vi "Actor Core.vi"(8 "error in":errorcluster, 11 "Panel Manager Controller.lvclass":refnum<class "Panel Manager Controller.lvclass">) -> (0 "error out":errorcluster, 3 "Actor out":refnum<class "Actor.lvclass">)   [LabVIEW 2015, in "Panel Manager Controller.lvclass"]
doc: "(<B>Filename</B>: Actor Framework.lvlib:Actor.lvclass:Actor Core.vi)\n\nReceives messages to the actor, reacts to them, and initiates any error handling that may shut the actor down.\n\nDescendant classes may override this VI to append parallel tasks for the actor to complete while it handles messages. Overrides use the Call Parent Method node."
uses:
  Panel Manager Controller.lvclass
  <vilib>/ActorFramework/Actor/Actor.lvclass
  Type Definition/Controls and VI Refnums.ctl
  Panel View/Panel View.lvclass
  Panel View/Panel View.lvclass/Panel View.ctl
  Panel Manager Controller.lvclass/Panel Manager Controller.ctl
  <vilib>/ActorFramework/Actor/Actor.lvclass/Actor.ctl
  <vilib>/ActorFramework/Message Enqueuer/Message Enqueuer.lvclass/Message Enqueuer.ctl
  <vilib>/ActorFramework/Stop Msg/Stop Msg.lvclass/Stop Msg.ctl
  Panel Manager Messages/Launch Panel Thread Msg/Launch New Panel Msg.lvclass/Launch New Panel Msg.ctl
  <vilib>/ActorFramework/Message Enqueuer/Init from Existing Queue.vi
  <vilib>/ActorFramework/Message Enqueuer/Enqueue Critical.vi
  <vilib>/ActorFramework/Message Enqueuer/Enqueue.vi
  <vilib>/ActorFramework/Message Priority Queue/Priority Enqueue.vi
  <vilib>/ActorFramework/Message Enqueuer/Message Enqueuer.lvclass
  <vilib>/ActorFramework/Stop Msg/Stop Msg.lvclass
  Panel Manager Messages/Launch Panel Thread Msg/Launch New Panel Msg.lvclass
  Panel Manager Messages/Insert Brower Panel Msg/Insert Brower Panel Msg.lvclass
panel:
  in  "Brower Insert":bool
  in  "Panel Insert":bool
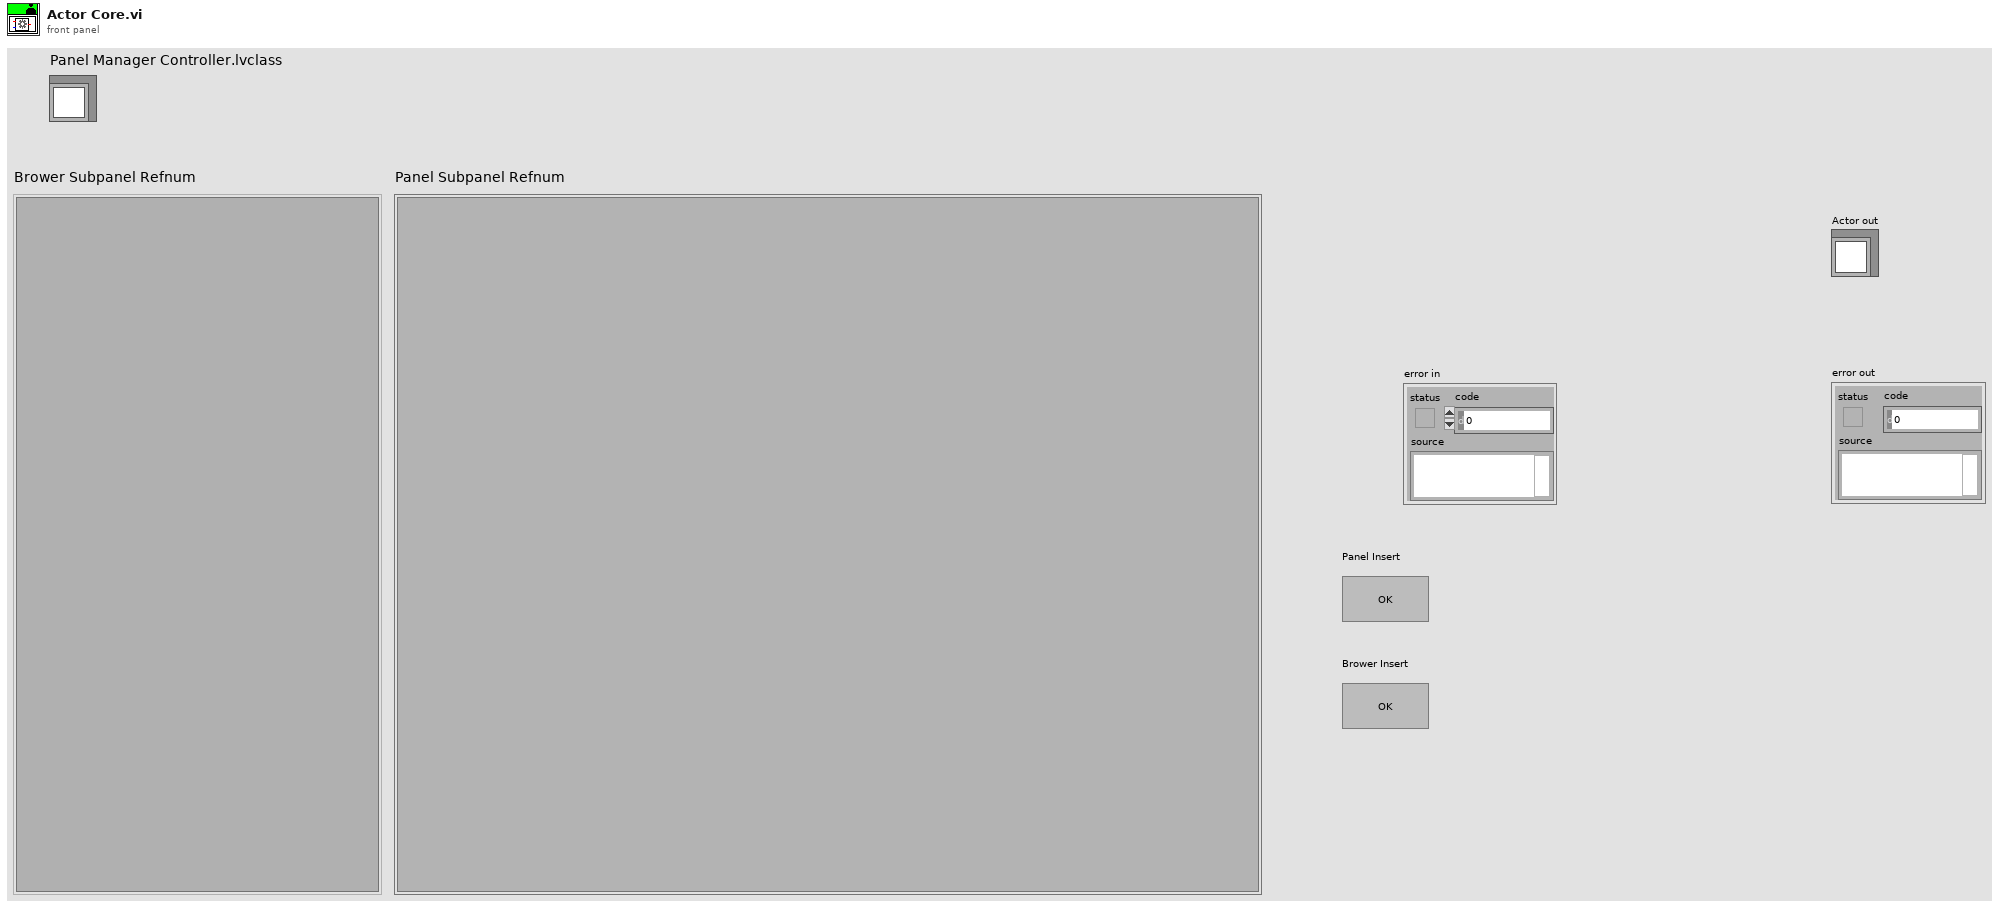
[diagram p1: front panel]
types:
  T1 = typedef "Panel Manager Controller.lvclass/Controls and VI Refnums.ctl" = cluster{"Panel Subpanel Refnum":refnum<vi>, "Brower Subpanel Refnum":refnum<vi>, "This VI":refnum<vi>}
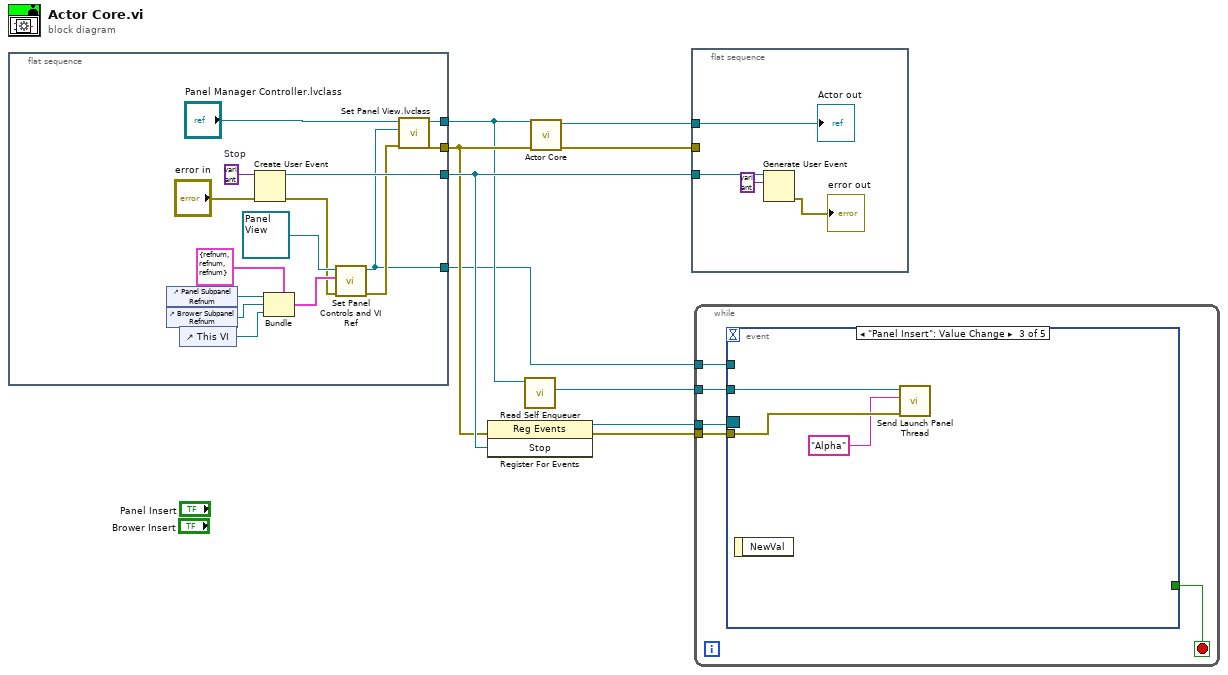
[diagram p0: block diagram]
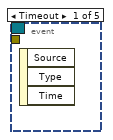
[diagram p2: hidden frame]
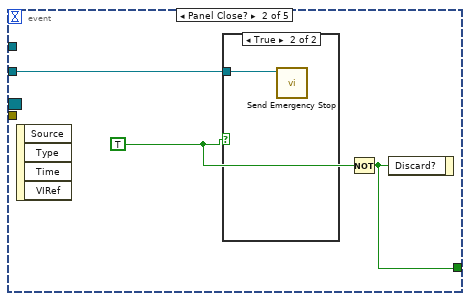
[diagram p3: hidden frame]
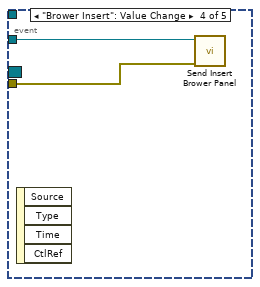
[diagram p5: hidden frame]
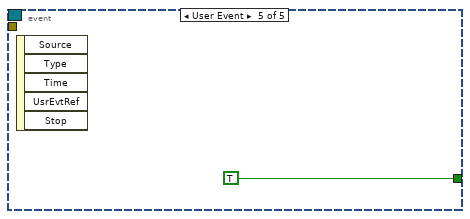
[diagram p6: hidden frame]
diagram:
  n1 = flat-sequence {
    tunnel: [w23] -> w6
    tunnel: [w15] -> w3
    tunnel: [w14] -> w2
    tunnel: [w13] -> w1
    frame #0 {
      w24 = variant  # Stop
      n2 = control-ref of="Panel Subpanel Refnum"() -> (w21:refnum<vi>)
      n3 = control-ref of="Brower Subpanel Refnum"() -> (w12:refnum<vi>)
      n4 = control-ref of="This VI"() -> (w11:refnum<vi>)
      n5 = Create User Event(user event datatype=w24, error in="error in") -> (user event=w23:refnum<user-event>, error out=w17:errorcluster)
      n6 = Bundle(cluster=T1 {"Panel Subpanel Refnum"=refnum, "Brower Subpanel Refnum"=refnum, "This VI"=refnum}, "Panel Subpanel Refnum"=w21, "Brower Subpanel Refnum"=w12, "This VI"=w11) -> (w18:T1)
      n7 = call "Set Panel Controls and VI Ref.vi"("error in (no error)"=w17, "Controls and VI Refnum"=w18, "Panel View.lvclass"=refnum<class "Panel View.lvclass"> refnum) -> ("error out"=w16:errorcluster, "Panel View.lvclass Out"=w13:refnum<class "Panel View.lvclass">)  [unwired: 7 in]
      n8 = call "Set Panel View.lvclass.vi"("error in (no error)"=w16, "Panel View.lvclass"=w13, "Panel Manager Controller.lvclass"="Panel Manager Controller.lvclass") -> ("error out"=w15:errorcluster, "Panel Manager Controller.lvclass out"=w14:refnum<class "Panel Manager Controller.lvclass">)  [unwired: 7 in]
    }
  }
  n9 = register-events(error in=w3, w6) -> (reference out=w7:refnum<event-registration>, error out=w8:errorcluster)  [unwired: 1 in]
  n10 = call <vilib>:"Read Self Enqueuer.vi"("Actor"=w2) -> ("Self Enqueuer"=w9:refnum<class "Message Enqueuer.lvclass">)  [unwired: 10 in]
  n11 = call-parent "Actor Core.vi"("error in"=w3, "Actor in"=w2) -> ("error out"=w4:errorcluster, "Actor out"=w5:refnum<class "Actor.lvclass">)  [unwired: 8 in]
  n12 = flat-sequence {
    tunnel: w6 -> [w28]
    tunnel: w5 -> [w25]
    tunnel: w4 -> [_]
    frame #0 {
      n13 = Generate User Event(user event=w28, event data cluster=variant ("event data")) -> (error out=→"error out":errorcluster)  [unwired: 2 in, 1 out]
      "Actor out" <- w25
    }
  }
  n14 = while {
    tunnel: w7 -> [w33]
    tunnel: w8 -> [w29]
    tunnel: w9 -> [w32]
    tunnel: w1 -> [w31]
    stop <- w30 stop-if-true
    n15 = event shown="[2] \"Panel Insert\": Value Change" {
      selector: w33 -> [_ _ _ _ _]
      dyn-events: _ -> [_ _ _ _ _]
      timeout: _ -> [_ _ _ _ _]
      tunnel: w32 -> [_ w36 w40 w42 _]
      tunnel: w31 -> [_ _ _ _ _]
      tunnel: [_ w34 _ _ TRUE] -> w30
      tunnel: w29 -> [_ _ w39 w41 _]
      event Timeout {
        n16 = event-data() -> ()  [unwired: 1 in, 3 out]
      }
      event Panel Close? {
        w35 = TRUE
        n17 = event-data() -> ()  [unwired: 1 in, 4 out]
        n18 = case shown="True" w35 {
          tunnel: w36 -> [_ w37]
          frame False {
          }
          frame True {
            n19 = call <vilib>:"Send Emergency Stop.vi"("Message Enqueuer"=w37) -> ()  [unwired: 10 in, 1 out]
          }
        }
        n20 = Not(x=w35) -> (.not. x?=w34:bool)
        n21 = event-data("Discard?"=w34) -> ()  [unwired: 1 in, 1 out]
      }
      event "Panel Insert": Value Change {
        n22 = event-data() -> ()  [unwired: 1 in, 1 out]
        n23 = call "Send Launch Panel Thread.vi"("error in (no error)"=w39, "Front Panel Window:Title(\"\")"="Alpha" ("Front Panel Window:Title(\"\")"), "Message Enqueuer"=w40) -> ()  [unwired: 7 in, 2 out]
      }
      event "Brower Insert": Value Change {
        n24 = event-data() -> ()  [unwired: 1 in, 4 out]
        n25 = call "Send Insert Brower Panel.vi"("error in (no error)"=w41, "Message Enqueuer"=w42) -> ()  [unwired: 8 in, 2 out]
      }
      event User Event {
        n26 = event-data() -> ()  [unwired: 1 in, 5 out]
      }
    }
  }
